vi "VisionConversions.vi"() -> ()   [LabVIEW 2019]
uses:
  sensors.vi
panel:
  in  "Offset":dbl=94.66
  out "Yaw":dbl
  out "Y":dbl
  out "X":dbl
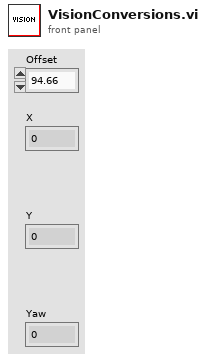
[diagram p1: front panel]
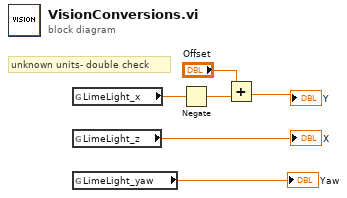
[diagram p0: block diagram]
diagram:
  # "unknown units- double check"
  n1 = global read "sensors.vi" "LimeLight_x"() -> (w5:dbl)
  n2 = global read "sensors.vi" "LimeLight_z"() -> (→"X":dbl)
  n3 = global read "sensors.vi" "LimeLight_yaw"() -> (→"Yaw":dbl)
  n4 = Negate(x=w5) -> (-x=w3:dbl)
  n5 = Add(x="Offset", y=w3) -> (x+y=→"Y":dbl)
